vi "balance grid.vi"(6 "init(0)":i32, 8 "Balance":bool, 9 "Device Addresses":refnum<visa-resource-name>[](array[refnum]), 10 "All Values":i32[][](array[numeric]), 11 "KW Values":i32[](array[numeric])) -> (1 "Load Balance":i32, 2 "Loads Requested":i32, 3 "Grid Power (KW)":i32, 4 "CO2 Accum":i32)   [LabVIEW 2024]
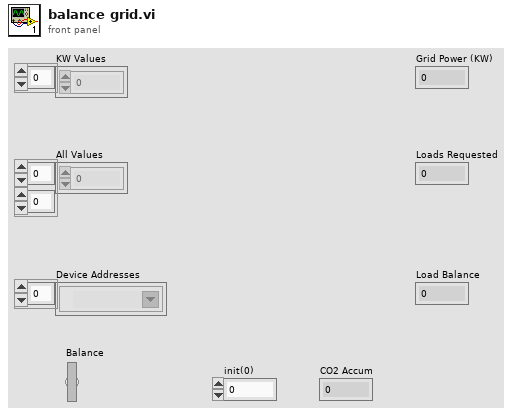
[diagram p1: front panel]
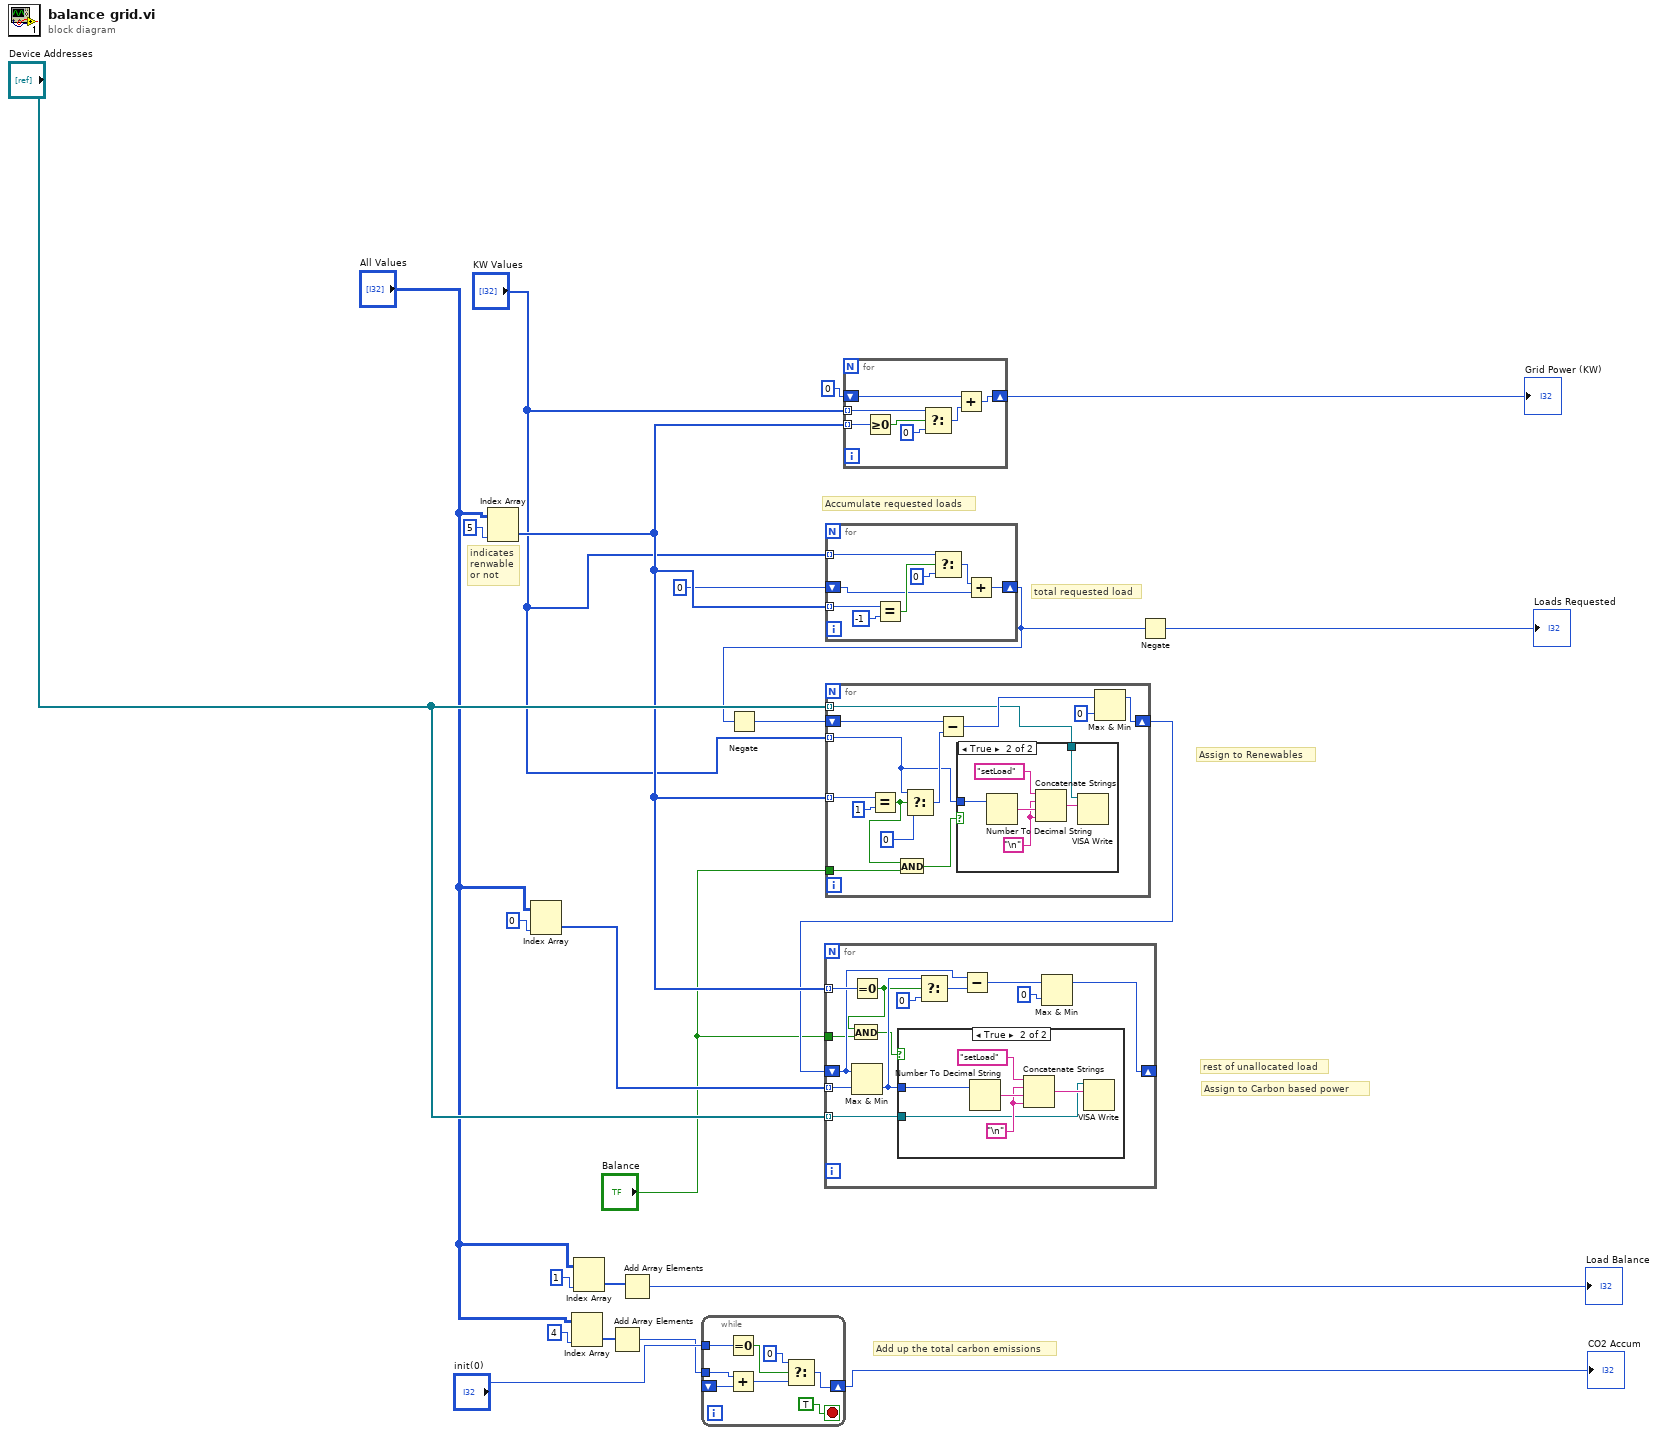
[diagram p0: block diagram]
diagram:
  # "indicates\nrenwable\nor not"
  # "Add up the total carbon emissions"
  # "Assign to Carbon based power"
  # "Assign to Renewables"
  # "rest of unallocated load"
  # "total requested load"
  # "Accumulate requested loads"
  n1 = Index Array(array="All Values", index (col)=5 ("disabled index (col)")) -> (element=w20:i32[])  [unwired: 1 in]
  n2 = Index Array(array="All Values", index (col)=0 ("disabled index (col)")) -> (element=w7:i32[])  [unwired: 1 in]
  n3 = Index Array(array="All Values", index (col)=4 ("disabled index (col)")) -> (element=w13:i32[])  [unwired: 1 in]
  n4 = Index Array(array="All Values", index (col)=1 ("disabled index (col)")) -> (element=w12:i32[])  [unwired: 1 in]
  n5 = Add Array Elements(numeric array=w13) -> (sum=w15:i32)
  n6 = Add Array Elements(numeric array=w12) -> (sum=→"Load Balance":i32)
  n7 = while {
    shift-right: [w24] -> w16
    shift-left: _ -> [w30]
    tunnel: w15 -> [w31]
    tunnel: "init(0)" -> [w29]
    stop <- TRUE stop-if-true
    n8 = Equal To 0?(x=w29) -> (x = 0?=w27:bool)
    n9 = Add(x=w31, y=w30) -> (x+y=w25:i32)
    n10 = Select(t=0, s=w27, f=w25) -> (s? t:f=w24:i32)
  }
  "CO2 Accum" <- w16
  n11 = for {
    tunnel: w20 -> [w39] mode=indexing
    shift-right: [w32] -> w9
    shift-left: 0 -> [w36]
    tunnel: "KW Values" -> [w35] mode=indexing
    n12 = Equal?(x=w39, y=-1) -> (x = y?=w37:bool)
    n13 = Select(t=w35, s=w37, f=0) -> (s? t:f=w34:i32)
    n14 = Add(x=w34, y=w36) -> (x+y=w32:i32)
  }
  n15 = Negate(x=w9) -> (-x=w8:i32)
  n16 = for {
    tunnel: w20 -> [w51] mode=indexing
    shift-right: [w46] -> w6
    shift-left: w8 -> [w50]
    tunnel: "KW Values" -> [w45] mode=indexing
    tunnel: "Device Addresses" -> [w44] mode=indexing
    tunnel: "Balance" -> [w41]
    n17 = Equal?(x=w51, y=1) -> (x = y?=w42:bool)
    n18 = And(x=w42, y=w41) -> (x .and. y?=w40:bool)
    n19 = Select(t=w45, s=w42, f=0) -> (s? t:f=w49:i32)
    n20 = Subtract(x=w50, y=w49) -> (x-y=w48:i32)
    n21 = case shown="True" w40 {
      tunnel: w45 -> [_ w56]
      tunnel: w44 -> [_ w53]
      frame False {
      }
      frame True {
        w54 = "\n"
        n22 = Number To Decimal String(number=w56) -> (decimal integer string=w57:string)  [unwired: 1 in]
        n23 = Concatenate Strings("setLoad" ("string"), w54, w57, w54) -> (w58:string)
        n24 = VISA Write(VISA resource name=w53, write buffer=w58) -> ()  [unwired: 1 in, 3 out]
      }
    }
    n25 = Max & Min(x=w48, y=0) -> (max(x,y)=w46:i32)  [unwired: 1 out]
  }
  n26 = for {
    tunnel: w20 -> [w69] mode=indexing
    shift-right: [w70] -> _
    shift-left: w6 -> [w67]
    tunnel: w7 -> [w68] mode=indexing
    tunnel: "Device Addresses" -> [w62] mode=indexing
    tunnel: "Balance" -> [w59]
    n27 = Equal To 0?(x=w69) -> (x = 0?=w60:bool)
    n28 = And(x=w60, y=w59) -> (x .and. y?=w61:bool)
    n29 = Max & Min(x=w67, y=w68) -> (min(x,y)=w64:i32)  [unwired: 1 out]
    n30 = case shown="True" w61 {
      tunnel: w64 -> [_ w74]
      tunnel: w62 -> [_ w72]
      frame False {
      }
      frame True {
        w75 = "\n"
        n31 = Number To Decimal String(number=w74) -> (decimal integer string=w76:string)  [unwired: 1 in]
        n32 = Concatenate Strings("setLoad" ("string"), w75, w76, w75) -> (w77:string)
        n33 = VISA Write(VISA resource name=w72, write buffer=w77) -> ()  [unwired: 1 in, 3 out]
      }
    }
    n34 = Select(t=w64, s=w60, f=0) -> (s? t:f=w63:i32)
    n35 = Subtract(x=w67, y=w63) -> (x-y=w66:i32)
    n36 = Max & Min(x=w66, y=0) -> (max(x,y)=w70:i32)  [unwired: 1 out]
  }
  n37 = for {
    tunnel: "KW Values" -> [w78] mode=indexing
    tunnel: w20 -> [w83] mode=indexing
    shift-right: [w80] -> w21
    shift-left: 0 -> [w81]
    n38 = Greater Or Equal To 0?(x=w83) -> (x >= 0?=w84:bool)
    n39 = Select(t=w78, s=w84, f=0) -> (s? t:f=w82:i32)
    n40 = Add(x=w81, y=w82) -> (x+y=w80:i32)
  }
  "Grid Power (KW)" <- w21
  n41 = Negate(x=w9) -> (-x=→"Loads Requested":i32)
